vi "Sign.vi"   [LabVIEW 2021]
uses:
  RSA/RSA.lvclass
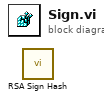
[diagram p0: block diagram]
diagram:
  n1 = call "RSA Sign Hash.vi"() -> ()  [unwired: 9 in, 3 out]
